vi "Query MSO and Number of Channels.vi"(8 "error in (no error)":errorcluster, 10 "Unit Info":T1) -> (0 "error out":errorcluster, 1 "No. Channels":i16, 2 "MSO?":bool)   [LabVIEW 2018, in "PicoScope 3000a.lvlib" / "PicoScope 3000a.lvclass"]
uses:
  PicoScope 3000a.lvclass
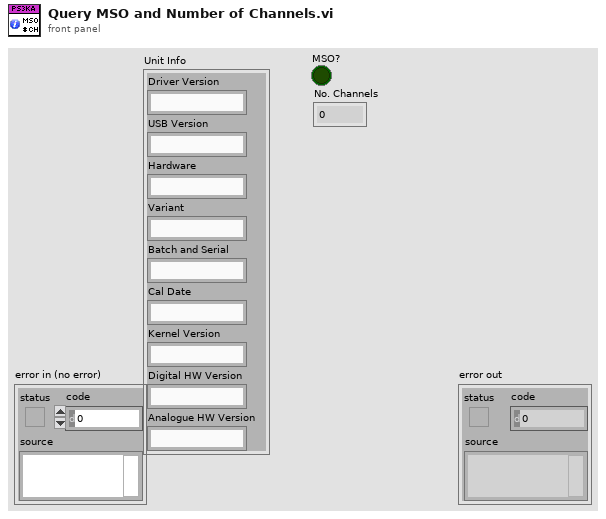
[diagram p1: front panel]
types:
  T1 = cluster{"Driver Version":string, "USB Version":string, "Hardware":string, "Variant":string, "Batch and Serial":string, "Cal Date":string, "Kernel Version":string, "Digital HW Version":string, "Analogue HW Version":string}
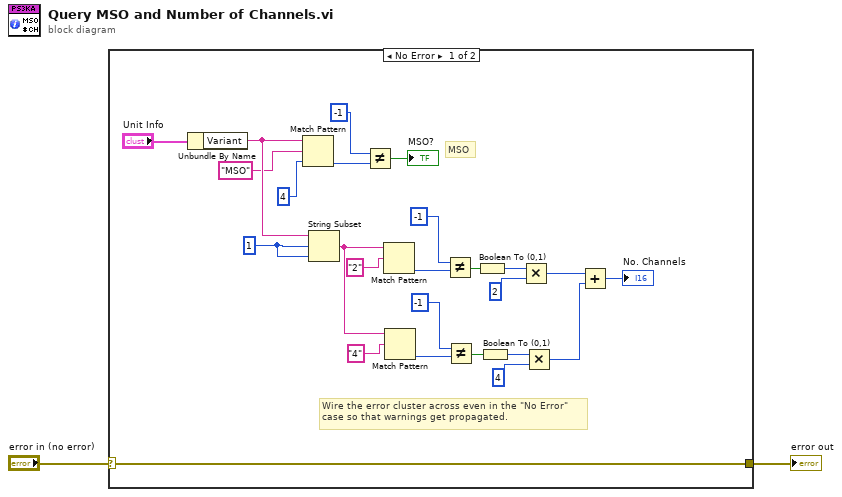
[diagram p0: block diagram]
diagram:
  n1 = case shown="No Error" "error in (no error)" {
    selector: "error in (no error)" -> [w27 w28]
    tunnel: [w27 w28] -> w1
    frame No Error {
      w26 = 1 ("offset (0)")
      # "MSO"
      # "Wire the error cluster across even in the \"No Error\"\ncase so that warnings get propagated."
      n2 = Unbundle By Name("Unit Info") -> ("Variant"=w22:string)
      n3 = Match Pattern(string=w22, regular expression="MSO", offset (0)=4) -> (offset past match=w19:i32)  [unwired: 3 out]
      n4 = String Subset(string=w22, offset (0)=w26, length (rest)=w26) -> (substring=w14:string)
      n5 = Not Equal?(x=-1, y=w19) -> (x != y?=→"MSO?":bool)
      n6 = Match Pattern(string=w14, regular expression="2") -> (offset past match=w24:i32)  [unwired: 1 in, 3 out]
      n7 = Match Pattern(string=w14, regular expression="4") -> (offset past match=w16:i32)  [unwired: 1 in, 3 out]
      n8 = Not Equal?(x=-1, y=w24) -> (x != y?=w11:bool)
      n9 = Not Equal?(x=-1, y=w16) -> (x != y?=w7:bool)
      n10 = Boolean To (0,1)(Boolean=w11) -> (0, 1=w10:i16)
      n11 = Boolean To (0,1)(Boolean=w7) -> (0, 1=w8:i16)
      n12 = Multiply(x=w10, y=i16 2) -> (x*y=w13:i16)
      n13 = Multiply(x=w8, y=i16 4) -> (x*y=w6:i16)
      n14 = Add(x=w13, y=w6) -> (x+y=→"No. Channels":i16)
    }
    frame Error {
    }
  }
  "error out" <- w1
